vi "InstrSwitch.vi"(0 "Bras_OUT":bool, 5 "instruments.ini":path=path "C:/BonOMM_git/Config/instruments.ini") -> (6 "This VI's Path":path, 13 "Code de fermeture":string, 14 "Instrument OUT":string, 15 "FoV":dbl caption="Champ de Vue" format="%.2g", 16 "foynom":i32 caption="Foyer nominale à 0°", 17 "atherm":dbl caption="Coefficient d'athermalisation" format="%.3g", 18 "exclusion":path caption="Chemin vers le fichier d'exclusion", 19 "collim":path caption="Chemin vers le fichier de collimation")   [LabVIEW 2019]
uses:
  <vilib>/Utility/config.llb/Read Key (String).vi
  <vilib>/Utility/config.llb/Read Key (Double).vi
  <vilib>/Utility/config.llb/Read Key (I32).vi
  <vilib>/Utility/config.llb/Read Key (Path).vi
  <vilib>/Utility/config.llb/Write Key (Boolean).vi
  <vilib>/Utility/config.llb/NI_LVConfig.lvlib
panel:
  out "Indicateur":string
  in  "Changer":bool
  in  "Annuler":bool
  out "Instrument Secondaire  IN":string
  out "Instrument Primaire  IN":string
  in  "ok":bool
  in  "?":i32(ring) items=["Pesto", "POMM", "CPAPIR", "Simon", "Spectro", "SpiOMM", "PANO-II+CCD4Kx4K", "CCD4Kx4K", "PANO-I+EMCCD", "POLARIMETRE"]
  # "[minutes d'arc]"
  # "[ADU]"
  # "[ADU/°K]"
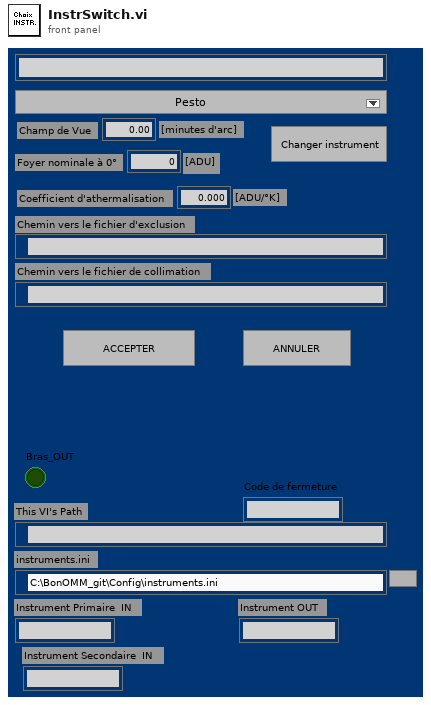
[diagram p1: front panel]
types:
  T1 = typedef "NI_LVConfig.lvlib/Config Data RefNum.ctl" = refnum<k1>
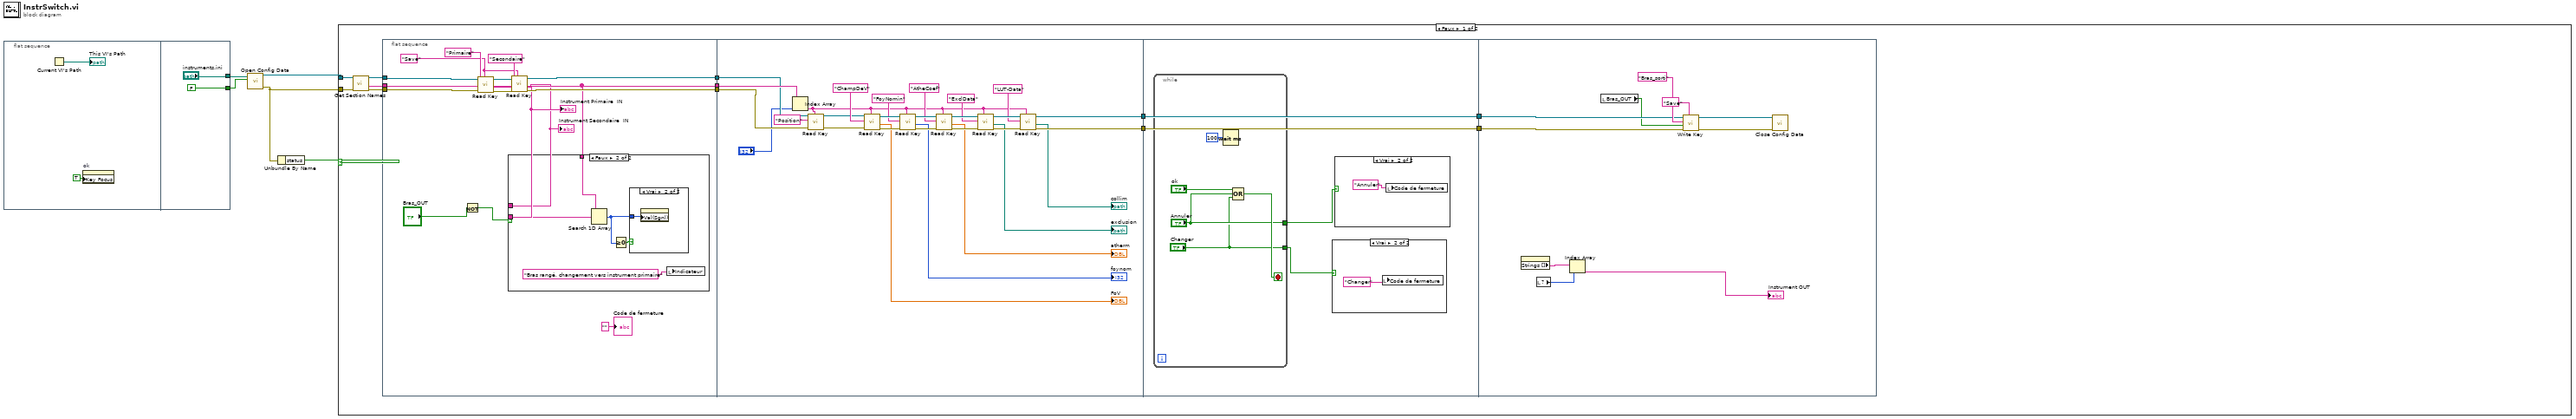
[diagram p0: block diagram]
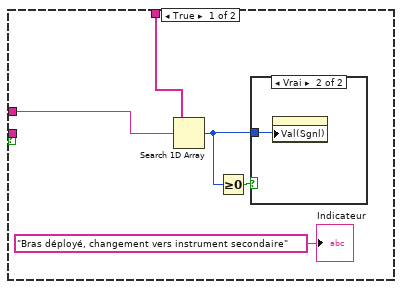
[diagram p2: hidden frame]
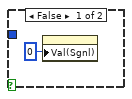
[diagram p3: hidden frame]
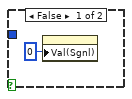
[diagram p4: hidden frame]
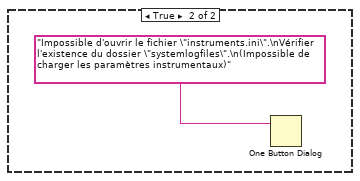
[diagram p7: hidden frame]
diagram:
  n1 = flat-sequence {
    tunnel: [FALSE ("create file if necessary (T)")] -> w5
    tunnel: ["instruments.ini"] -> w1
    frame #0 {
      n2 = Current VI's Path() -> (path=→"This VI's Path":path)
      n3 = property on="ok" class="Bool"("Key Focus"=TRUE) -> ()  [unwired: 2 in, 2 out]
    }
    frame #1 {
    }
  }
  n4 = call <vilib>:"Open Config Data.vi"("create file if necessary (T)"=w5, "configuration file path"=w1) -> ("error out"=w3:errorcluster, "refnum"=w4:T1)  [unwired: 7 in, 1 out]
  n5 = Unbundle By Name(w3) -> ("status"=w2:bool)
  n6 = case shown="Faux" w2 {
    tunnel: w4 -> [w21 _]
    tunnel: w3 -> [w20 _]
    frame False {
      n7 = call <vilib>:"Get Section Names.vi"("error in (no error)"=w20, "refnum"=w21) -> ("error out"=w17:errorcluster, "section names"=w18:string[], "refnum out"=w19:T1)  [unwired: 7 in]
      n8 = flat-sequence {
        tunnel: w19 -> [w27]
        tunnel: w18 -> [w29]
        tunnel: [w31] -> w16
        tunnel: w17 -> [w26]
        tunnel: [w34] -> w15
        tunnel: [w29] -> w14
        tunnel: w16 -> [w76]
        tunnel: w15 -> [w77]
        tunnel: w14 -> [w78]
        tunnel: [w75] -> w13
        tunnel: [w74] -> w11
        tunnel: w13 -> [w82]
        tunnel: [w82] -> w12
        tunnel: w11 -> [w81]
        tunnel: [w81] -> w10
        tunnel: w12 -> [w93]
        tunnel: w10 -> [w92]
        frame #0 {
          w28 = "Save" ("section")
          n9 = Not(x="Bras_OUT") -> (.not. x?=w23:bool)
          n10 = call-poly <vilib>:"Read Key.vi"("section"=w28, "error in (no error)"=w26, "key"="Primaire", "refnum"=w27) -> ("error out"=w32:errorcluster, "value"=w30:string, "refnum out"=w35:T1)  [unwired: 4 in, 1 out]
          "Instrument Primaire  IN" <- w30
          n11 = call-poly <vilib>:"Read Key.vi"("section"=w28, "error in (no error)"=w32, "key"="Secondaire", "refnum"=w35) -> ("error out"=w31:errorcluster, "value"=w25:string, "refnum out"=w34:T1)  [unwired: 4 in, 1 out]
          "Instrument Secondaire  IN" <- w25
          n12 = case shown="Faux" w23 {
            tunnel: w30 -> [_ w46]
            tunnel: w29 -> [w39 w45]
            tunnel: w25 -> [w38 _]
            frame True {
              n13 = Search 1D Array(1D array=w39, element=w38) -> (index of element=w40:i32)  [unwired: 1 in]
              n14 = Greater Or Equal To 0?(x=w40) -> (x >= 0?=w41:bool)
              n15 = case shown="Vrai" w41 {
                tunnel: w40 -> [_ w43]
                frame False {
                  n16 = property class="MDér (strict)"("Val(Sgnl)"=0) -> ()  [unwired: 2 in, 2 out]
                }
                frame True {
                  n17 = property class="MDér (strict)"("Val(Sgnl)"=w43) -> ()  [unwired: 2 in, 2 out]
                }
              }
              "Indicateur" <- "Bras déployé, changement vers instrument secondaire" ("Chaîne")
            }
            frame False {
              n18 = Search 1D Array(1D array=w45, element=w46) -> (index of element=w47:i32)  [unwired: 1 in]
              n19 = Greater Or Equal To 0?(x=w47) -> (x >= 0?=w48:bool)
              n20 = case shown="Vrai" w48 {
                tunnel: w47 -> [_ w50]
                frame False {
                  n21 = property class="MDér (strict)"("Val(Sgnl)"=0) -> ()  [unwired: 2 in, 2 out]
                }
                frame True {
                  n22 = property class="MDér (strict)"("Val(Sgnl)"=w50) -> ()  [unwired: 2 in, 2 out]
                }
              }
              n23 = local write "Indicateur"("Bras rangé, changement vers instrument primaire" ("Chaîne")) -> ()
            }
          }
          "Code de fermeture" <- "" ("Chaîne")
        }
        frame #1 {
          n24 = Index Array(array=w78, index="?") -> (element=w53:string)
          n25 = call-poly <vilib>:"Read Key.vi"("section"=w53, "error in (no error)"=w76, "key"="Position", "refnum"=w77) -> ("error out"=w52:errorcluster, "refnum out"=w54:T1)  [unwired: 4 in, 2 out]
          n26 = call-poly <vilib>:"Read Key.vi"("section"=w53, "error in (no error)"=w52, "key"="ChampDeV", "refnum"=w54) -> ("error out"=w71:errorcluster, "value"=→"FoV":dbl, "refnum out"=w72:T1)  [unwired: 4 in, 1 out]
          n27 = call-poly <vilib>:"Read Key.vi"("section"=w53, "error in (no error)"=w71, "key"="FoyNomin", "refnum"=w72) -> ("error out"=w69:errorcluster, "value"=→"foynom":i32, "refnum out"=w70:T1)  [unwired: 4 in, 1 out]
          n28 = call-poly <vilib>:"Read Key.vi"("section"=w53, "error in (no error)"=w69, "key"="AtheCoef", "refnum"=w70) -> ("error out"=w65:errorcluster, "value"=→"atherm":dbl, "refnum out"=w66:T1)  [unwired: 4 in, 1 out]
          n29 = call-poly <vilib>:"Read Key.vi"("section"=w53, "error in (no error)"=w65, "key"="ExclData", "refnum"=w66) -> ("error out"=w68:errorcluster, "value"=→"exclusion":path, "refnum out"=w67:T1)  [unwired: 4 in, 1 out]
          n30 = call-poly <vilib>:"Read Key.vi"("section"=w53, "error in (no error)"=w68, "key"="LUT-Data", "refnum"=w67) -> ("error out"=w74:errorcluster, "value"=→"collim":path, "refnum out"=w75:T1)  [unwired: 4 in, 1 out]
        }
        frame #2 {
          n31 = while {
            tunnel: ["Annuler"] -> w80
            tunnel: ["Changer"] -> w79
            stop <- w87 stop-if-true
            n32 = Wait (ms)(milliseconds to wait=u32 100 ("attente (ms)")) -> ()  [unwired: 1 out]
            n33 = Compound Arithmetic op=OR ("Opérateur arithmétique")("ok", "Annuler", "Changer") -> (w87:bool)
          }
          n34 = case shown="Vrai" w79 {
            frame False {
            }
            frame True {
              n35 = local write "Code de fermeture"("Changer") -> ()
            }
          }
          n36 = case shown="Vrai" w80 {
            frame False {
            }
            frame True {
              n37 = local write "Code de fermeture"("Annuler") -> ()
            }
          }
        }
        frame #3 {
          n38 = property class="MDér (strict)"() -> ("Strings []"=w95:string[])  [unwired: 2 in, 2 out]
          n39 = local read item#1() -> (w96:i32)
          n40 = Index Array(array=w95, index=w96) -> (element=→"Instrument OUT":string)
          n41 = local read "Bras_OUT"() -> (w91:bool)
          n42 = call-poly <vilib>:"Write Key.vi"("section"="Save", "error in (no error)"=w92, "value"=w91, "key"="Bras_sorti", "refnum"=w93) -> ("error out"=w97:errorcluster, "refnum out"=w98:T1)  [unwired: 4 in, 1 out]
          n43 = call <vilib>:"Close Config Data.vi"("error in (no error)"=w97, "refnum"=w98) -> ()  [unwired: 8 in, 2 out]
        }
      }
    }
    frame True {
      n44 = One Button Dialog(message="Impossible d'ouvrir le fichier \"instruments.ini\".\nVérifier l'existence du dossier \"systemlogfiles\".\n(Impossible de charger les paramètres instrumentaux)") -> ()  [unwired: 1 in, 1 out]
    }
  }
